vi "Knock Read.vi"(6 "FIFO Indexes.Read":cluster{"Knock":i32[], "Knock Intensity":i32[]}={"Knock"=[-1, -1, -1, -1, -1, -1, -1, -1, -1, -1, -1, -1, -1, -1, -1, -1], "Knock Intensity"=[-1, -1, -1, -1, -1, -1, -1, -1, -1, -1, -1, -1, -1, -1, -1, -1]}, 7 "Device Outputs in":dbl[](array[numeric]), 10 "Knock Intensity":sgl[](array[numeric])=[0.0, 0.0, 0.0, 0.0, 0.0, 0.0, 0.0, 0.0, 0.0, 0.0, 0.0, 0.0, 0.0, 0.0, 0.0, 0.0], 11 "Knock":bool[](array[boolean])=[FALSE, FALSE, FALSE, FALSE, FALSE, FALSE, FALSE, FALSE, FALSE, FALSE, FALSE, FALSE, FALSE, FALSE, FALSE, FALSE]) -> (5 "Device Outputs out":dbl[](array[numeric]))   [LabVIEW 2016, in "DCM Engine.lvlib"]
uses:
  DCM Engine.lvlib
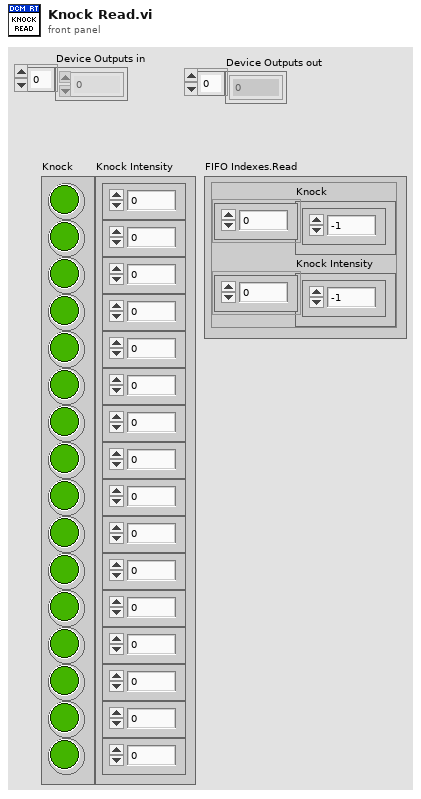
[diagram p1: front panel]
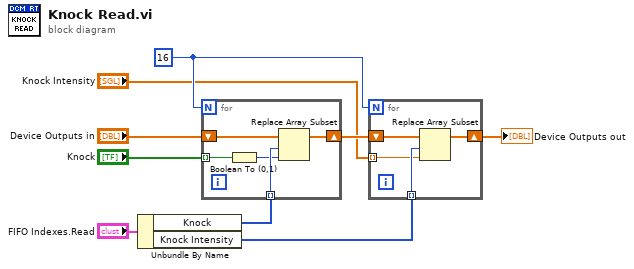
[diagram p0: block diagram]
diagram:
  w4 = 16
  n1 = Unbundle By Name("FIFO Indexes.Read") -> ("Knock"=w8:i32[], "Knock Intensity"=w5:i32[])
  n2 = for {
    N: w4 -> [_]
    shift-right: [w13] -> w7
    shift-left: "Device Outputs in" -> [w14]
    tunnel: "Knock" -> [w11] mode=indexing
    tunnel: w8 -> [w12] mode=indexing
    n3 = Boolean To (0,1)(Boolean=w11) -> (0, 1=w10:i16)
    n4 = Replace Array Subset(array=w14, new element=w10, index=w12) -> (w13:dbl[])
  }
  n5 = for {
    N: w4 -> [_]
    shift-right: [w17] -> w6
    shift-left: w7 -> [w18]
    tunnel: "Knock Intensity" -> [w15] mode=indexing
    tunnel: w5 -> [w16] mode=indexing
    n6 = Replace Array Subset(array=w18, new element=w15, index=w16) -> (w17:dbl[])
  }
  "Device Outputs out" <- w6
